vi "BCtr_Init.vi"(6 "BaseAddr":u16 format="%x", 7 "SBPort":string, 8 "error in (no error)":errorcluster, 9 "NC":u32 max=16777215 step=1, 10 "NB":u16[](array[numeric]), 11 "NA":u16[](array[numeric])) -> (0 "error out":errorcluster, 3 "CtrCfg":T1 {"BaseAddrOut" format="%x"})   [LabVIEW 2016]
uses:
  <vilib>/ErrorRing/Error Ring.xnode
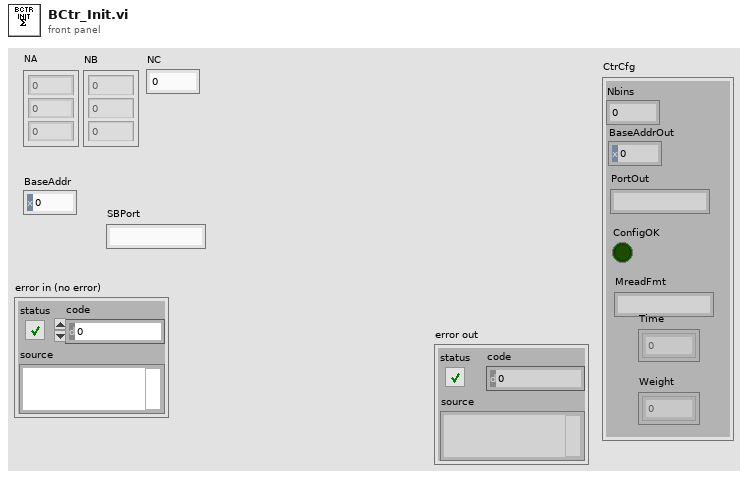
[diagram p1: front panel]
types:
  T1 = cluster{"Nbins":u16, "BaseAddrOut":u16, "PortOut":string, "ConfigOK":bool, "MreadFmt":string, "Time":dbl[], "Weight":dbl[]}
  T2 = cluster{u16, "BaseAddr":u16, "PortOut":string, bool, string, "T\nT":dbl[], "W":dbl[]}
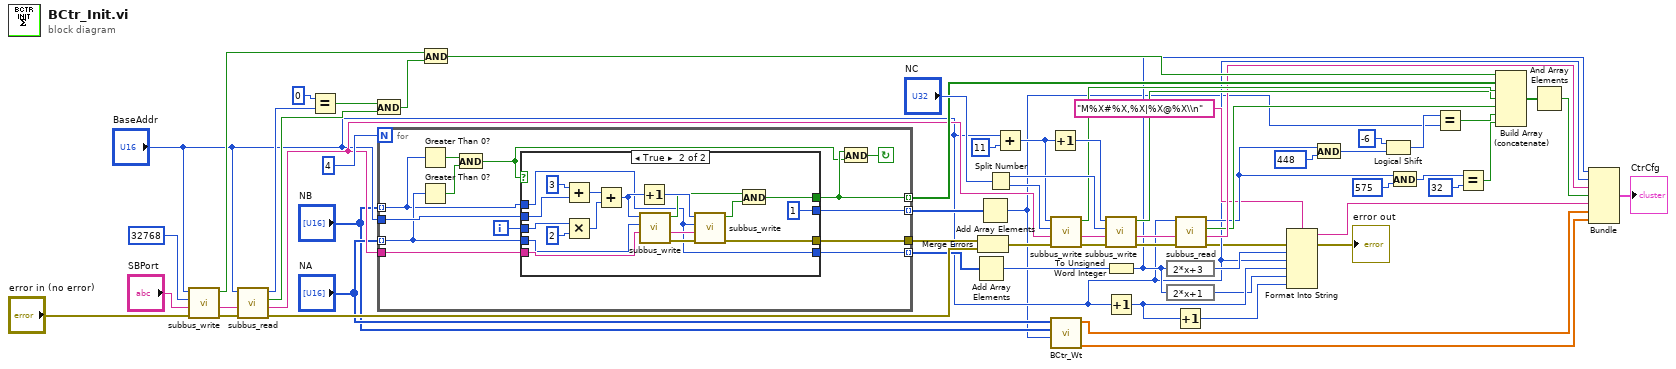
[diagram p0: block diagram]
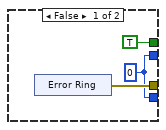
[diagram p2: hidden frame]
diagram:
  n1 = call "subbus_write.vi"("error in (no error)"="error in (no error)", "PortIn"="SBPort", "Data"=u16 32768, "Address"="BaseAddr") -> ("error out"=w57:errorcluster, "PortOut"=w58:string, "Ack"=w51:bool)  [unwired: 5 in]
  n2 = call "subbus_read.vi"("error in (no error)"=w57, "PortIn"=w58, "Address"="BaseAddr") -> ("error out"=w19:errorcluster, "PortOut"=w17:string, "Ack"=w53:bool, "Data"=w56:u16)  [unwired: 5 in]
  n3 = Equal?(x=0, y=w56) -> (x = y?=w54:bool)
  n4 = And(x=w54, y=w53) -> (x .and. y?=w52:bool)
  n5 = for {
    N: 4 -> [_]
    tunnel: "NA" -> [w72] mode=indexing
    tunnel: "NB" -> [w66] mode=indexing
    tunnel: w17 -> [w76]
    tunnel: "BaseAddr" -> [w74]
    tunnel: [w73] -> w20
    tunnel: [w69] -> w45 mode=indexing
    tunnel: [w64] -> w37 mode=indexing
    tunnel: [w65] -> w16 mode=indexing
    i -> [w75]
    stop <- w68 continue-if-true
    n6 = Greater Than 0?(x=w66) -> (x > 0?=w71:bool)
    n7 = Greater Than 0?(x=w72) -> (x > 0?=w70:bool)
    n8 = And(x=w71, y=w70) -> (x .and. y?=w67:bool)
    n9 = case shown="True" w67 {
      tunnel: w76 -> [_ w98]
      tunnel: w75 -> [_ w97]
      tunnel: w74 -> [_ w96]
      tunnel: [w78 w95] -> w73
      tunnel: w72 -> [_ w94]
      tunnel: [TRUE w93] -> w69
      tunnel: w66 -> [_ w82]
      tunnel: [w77 w82] -> w65
      tunnel: [w77 1] -> w64
      frame False {
        w77 = 0
        n10 = xnode "Error Ring"() -> ("error out"=w78:errorcluster)
      }
      frame True {
        n11 = Add(x=3, y=w96) -> (x+y=w88:i32)
        n12 = Multiply(x=w97, y=2) -> (x*y=w87:i32)
        n13 = Add(x=w88, y=w87) -> (x+y=w86:i32)
        n14 = Increment(x=w86) -> (x+1=w85:i32)
        n15 = call "subbus_write.vi"("PortIn"=w98, "Data"=w94, "Address"=w86) -> ("error out"=w92:errorcluster, "PortOut"=w91:string, "Ack"=w84:bool)  [unwired: 6 in]
        n16 = call "subbus_write.vi"("error in (no error)"=w92, "PortIn"=w91, "Data"=w82, "Address"=w85) -> ("error out"=w95:errorcluster, "Ack"=w83:bool)  [unwired: 5 in, 1 out]
        n17 = And(x=w84, y=w83) -> (x .and. y?=w93:bool)
      }
    }
    n18 = And(x=w69, y=w67) -> (x .and. y?=w68:bool)
  }
  n19 = And(x=w51, y=w52) -> (x .and. y?=w40:bool)
  n20 = Add Array Elements(numeric array=w16) -> (sum=w36:i32)
  n21 = Merge Errors(w20, w19) -> (w18:errorcluster)
  n22 = Add Array Elements(numeric array=w37) -> (sum=w3:i32)
  n23 = Split Number(x="NC") -> (hi(x)=w61:u16, lo(x)=w60:u16)
  n24 = Add(x="BaseAddr", y=11) -> (x+y=w49:i32)
  n25 = Increment(x=w49) -> (x+1=w46:i32)
  n26 = call "subbus_write.vi"("error in (no error)"=w18, "PortIn"=w17, "Data"=w60, "Address"=w49) -> ("error out"=w47:errorcluster, "PortOut"=w48:string, "Ack"=w44:bool)  [unwired: 5 in]
  n27 = call "BCtr_Wt.vi"("N_NAB"=w3, "NB"="NB", "NA"="NA") -> ("W"=w1:dbl[], "T\nT"=w2:dbl[])  [unwired: 7 in]
  n28 = call "subbus_write.vi"("error in (no error)"=w47, "PortIn"=w48, "Data"=w61, "Address"=w46) -> ("error out"=w33:errorcluster, "PortOut"=w35:string, "Ack"=w43:bool)  [unwired: 5 in]
  n29 = To Unsigned Word Integer(number=w36) -> (unsigned 16bit integer=w10:u16)
  n30 = Increment(x="BaseAddr") -> (x+1=w13:u16)
  n31 = expression code="2*x+3"(w10) -> (w14:u16)
  n32 = expression code="2*x+1"(w10) -> (w11:u16)
  n33 = Increment(x=w13) -> (x+1=w12:u16)
  n34 = call "subbus_read.vi"("error in (no error)"=w33, "PortIn"=w35, "Address"="BaseAddr") -> ("error out"=w8:errorcluster, "PortOut"=w34:string, "Ack"=w32:bool, "Data"=w27:u16)  [unwired: 5 in]
  n35 = Format Into String(format string="M%X#%X,%X|%X@%X\\n", error in=w8, w14, "BaseAddr", w13, w11, w12) -> (resulting string=w6:string, error out=→"error out":errorcluster)  [unwired: 1 in]
  n36 = And(x=w27, y=u16 448) -> (x .and. y?=w30:u16)
  n37 = Logical Shift(y=-6, x=w30) -> (x << y=w28:u16)
  n38 = And(x=w27, y=u16 575) -> (x .and. y?=w25:u16)
  n39 = Equal?(x=w28, y=w3) -> (x = y?=w23:bool)
  n40 = Equal?(x=w25, y=u16 32) -> (x = y?=w22:bool)
  n41 = Build Array (concatenate)(w40, w45, w44, w43, w32, w23, w22) -> (w42:bool[])
  n42 = And Array Elements(Boolean array=w42) -> (logical AND=w41:bool)
  n43 = Bundle(w10, "BaseAddr"="BaseAddr", "PortOut"=w34, w41, w6, "T\nT"=w2, "W"=w1) -> (→"CtrCfg":T2)  [unwired: 1 in]
